vi "ContextManager.FGV.vi"(10 "error in":errorcluster, 11 "action":T1) -> (2 "error out":errorcluster, 3 "context":refnum<class "zmq_context.lvclass">)   [LabVIEW 2019, in "RemoteControl.ZMQ.lvlib" / "ZMQ.ContextManager.lvlib"]
uses:
  ZMQ.ContextManager.lvlib
  <vilib>/addons/zeromq/zmq_context.lvclass
  Action--enum.ctl
panel:
  out "counter":u32
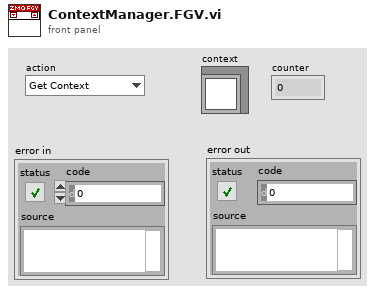
[diagram p1: front panel]
types:
  T1 = typedef "RemoteControl.ZMQ.lvlib/ZMQ.ContextManager.lvlib/Action--enum.ctl" = enum16{"Get Context", "Release Context", "Force Cleanup"}
  T2 = typedef "RemoteControl.ZMQ.lvlib/ZMQ.ContextManager.lvlib/Context--DVR.ctl" = refnum<data-value>
  T3 = typedef "RemoteControl.ZMQ.lvlib/ZMQ.ContextManager.lvlib/Context--Cluster.ctl" = cluster{"context":refnum<class "zmq_context.lvclass">, "counter":u32}
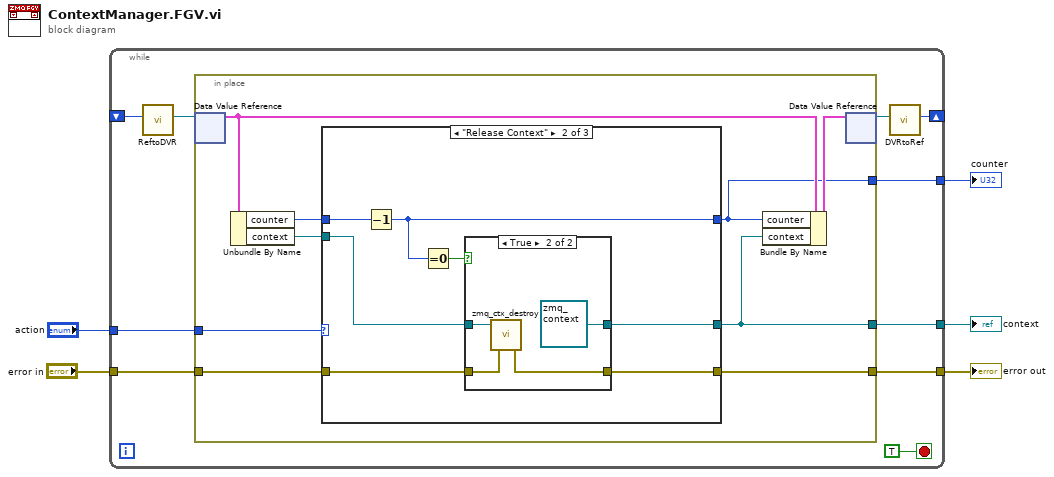
[diagram p0: block diagram]
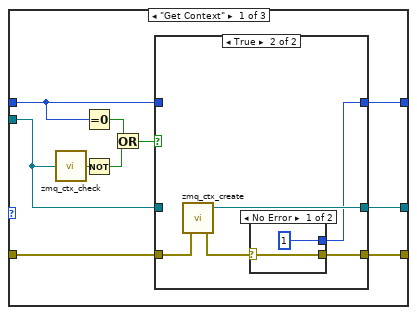
[diagram p2: hidden frame]
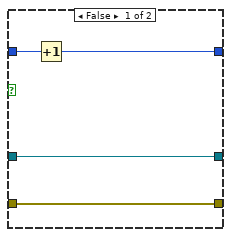
[diagram p3: hidden frame]
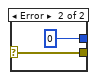
[diagram p4: hidden frame]
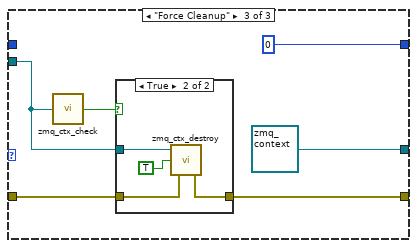
[diagram p6: hidden frame]
diagram:
  n1 = while {
    tunnel: "error in" -> [w10]
    tunnel: [w14] -> w4
    tunnel: "action" -> [w13]
    shift-right: [w8] -> _
    shift-left: _ -> [w11]
    tunnel: [w12] -> w3
    tunnel: [w6] -> w1
    stop <- TRUE stop-if-true
    n2 = call "ReftoDVR.vi"("Ref"=w11) -> ("DVR"=w7:T2)  [unwired: 10 in]
    n3 = in-place {
      in-place-border: w10 -> [w24]
      in-place-border: [w23] -> w14
      in-place-border: w13 -> [w22]
      in-place-border: [w18] -> w12
      in-place-border: [w16] -> w6
      n4 = in-place-dvr #1(w7) -> (w20:T3)  [unwired: 1 out]
      n5 = Unbundle By Name(w20) -> ("counter"=w17:u32, "context"=w21:refnum<class "zmq_context.lvclass">)
      n6 = case shown="\"Release Context\"" w22 {
        tunnel: w21 -> [w25 w48 w62]
        tunnel: [w32 w52 refnum<class "zmq_context.lvclass"> refnum ("context out")] -> w18
        tunnel: w24 -> [w34 w54 w66]
        tunnel: [w33 w53 w65] -> w23
        tunnel: w17 -> [w29 w51 _]
        tunnel: [w28 w50 u32 0] -> w16
        frame "Get Context" {
          n7 = call <vilib>:"zmq_ctx_check.vi"("context in"=w25) -> ("valid?"=w31:bool)
          n8 = Equal To 0?(x=w29) -> (x = 0?=w27:bool)
          n9 = Not(x=w31) -> (.not. x?=w26:bool)
          n10 = Or(x=w27, y=w26) -> (x .or. y?=w30:bool)
          n11 = case shown="True" w30 {
            tunnel: [w37 w43] -> w32
            tunnel: w34 -> [w38 w42]
            tunnel: [w38 w39] -> w33
            tunnel: w25 -> [w37 _]
            tunnel: w29 -> [w36 _]
            tunnel: [w35 w41] -> w28
            frame False {
              n12 = Increment(x=w36) -> (x+1=w35:u32)
            }
            frame True {
              n13 = call <vilib>:"zmq_ctx_create.vi"("error in"=w42) -> ("error out"=w40:errorcluster, "context out"=w43:refnum<class "zmq_context.lvclass">)  [unwired: 3 in]
              n14 = case shown="No Error" w40 {
                selector: w40 -> [w44 w46]
                tunnel: [u32 1 u32 0] -> w41
                tunnel: [w44 w46] -> w39
                frame No Error {
                }
                frame Error {
                }
              }
            }
          }
        }
        frame "Release Context" {
          n15 = Decrement(x=w51) -> (x-1=w50:u32)
          n16 = Equal To 0?(x=w50) -> (x = 0?=w49:bool)
          n17 = case shown="True" w49 {
            tunnel: w54 -> [w55 w60]
            tunnel: [w55 w59] -> w53
            tunnel: [w56 refnum<class "zmq_context.lvclass"> refnum ("context out")] -> w52
            tunnel: w48 -> [w56 w57]
            frame False {
            }
            frame True {
              n18 = call <vilib>:"zmq_ctx_destroy.vi"("error in"=w60, "context in"=w57) -> ("error out"=w59:errorcluster)  [unwired: 3 in]
            }
          }
        }
        frame "Force Cleanup" {
          n19 = call <vilib>:"zmq_ctx_check.vi"("context in"=w62) -> ("valid?"=w61:bool)
          n20 = case shown="True" w61 {
            tunnel: w66 -> [w67 w71]
            tunnel: [w67 w70] -> w65
            tunnel: w62 -> [_ w68]
            frame False {
            }
            frame True {
              n21 = call <vilib>:"zmq_ctx_destroy.vi"("error in"=w71, "reap? (F)"=TRUE, "context in"=w68) -> ("error out"=w70:errorcluster)  [unwired: 2 in]
            }
          }
        }
      }
      n22 = Bundle By Name(cluster=w20, "counter"=w16, "context"=w18) -> (w19:T3)
      n23 = in-place-dvr #1(w19) -> (w9:T2)  [unwired: 1 out]
    }
    n24 = call "DVRtoRef.vi"("DVR"=w9) -> ("Ref"=w8:u32)  [unwired: 10 in]
  }
  "context" <- w3
  "error out" <- w4
  "counter" <- w1
